vi "Do.vi"(8 "error in (no error)":errorcluster, 10 "Actor in":refnum<class "Actor.lvclass">, 11 "Update Bool Array":refnum<class "Update Bool Array.lvclass">) -> (0 "error out":errorcluster, 2 "Actor out":refnum<class "Actor.lvclass">)   [LabVIEW 2014, in "Update Bool Array.lvclass"]
doc: "(<B>Filename</B>: Actor Framework.lvlib:Message.lvclass:Do.vi)\n\nDefines what a message does when it is received by an actor. Generally, a message instructs an actor to invoke one of its methods. By default, this method does nothing. A child class must override it to define behavior. Create a child class by using the Actor Framework Message Maker dialog box."
uses:
  Update Bool Array.lvclass
  <vilib>/ActorFramework/Actor/Actor.lvclass
  Update Setting.lvclass/Update Setting.ctl
  Update Bool Array.lvclass/Update Bool Array.ctl
  <vilib>/NI/Current Value Table/DataTypes/Array of Boolean_Write.vi
  Read Key.vi
  Read Setting.vi
  <vilib>/NI/Current Value Table/Type to Enum.vi
  <vilib>/NI/Current Value Table/DataTypes/Array of Boolean_Type To Enum.vi
  <vilib>/NI/Current Value Table/Memory Block.vi
  <vilib>/NI/Current Value Table/DataTypes/Array of Boolean_Memory Block.vi
  <vilib>/NI/Current Value Table/FGVs/Tag Memory.vi
  <vilib>/NI/Current Value Table/FGVs/CVT Globals.vi
  <vilib>/NI/Current Value Table/Current Value Table.lvlib
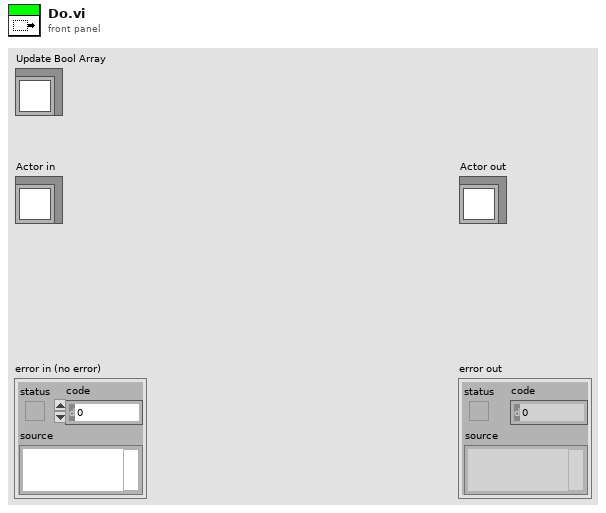
[diagram p1: front panel]
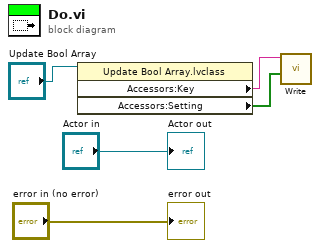
[diagram p0: block diagram]
diagram:
  n1 = property class="Update Bool Array.lvclass"(reference="Update Bool Array") -> ("Accessors:Key"=w2:string, "Accessors:Setting"=w1:bool[])  [unwired: 1 in, 2 out]
  n2 = call-poly <vilib>:"Write.vi"("Value"=w1, "Tag Name"=w2) -> ()  [unwired: 9 in, 1 out]
  "error out" <- "error in (no error)"
  "Actor out" <- "Actor in"
